vi "Constructor.vi"(6 "channel name":string, 8 "error in":errorcluster, 9 "group name":string, 10 "path":path, 11 "TDMS in":refnum<class "TDMS.lvclass">) -> (0 "error out":errorcluster, 3 "TDMS out":refnum<class "TDMS.lvclass">)   [LabVIEW 2011, in "TDMS.lvclass"]
uses:
  TDMS.lvclass
  TDMS.lvclass/TDMS.ctl
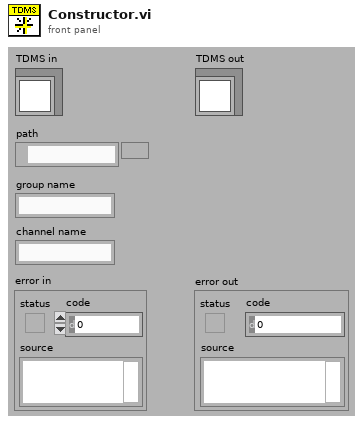
[diagram p1: front panel]
types:
  T1 = enum16{"open", "open or create", "create or replace", "create", "open (read-only)"}
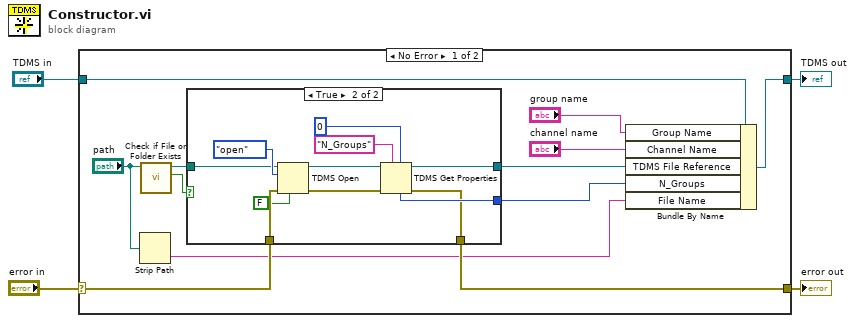
[diagram p0: block diagram]
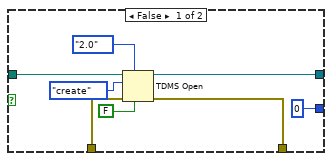
[diagram p2: hidden frame]
diagram:
  n1 = case shown="No Error" "error in" {
    selector: "error in" -> [w16 w37]
    tunnel: [w15 w37] -> w1
    tunnel: [w12 w36] -> w2
    tunnel: "TDMS in" -> [w14 w36]
    frame No Error {
      n2 = Strip Path(path="path") -> (name=w5:string)  [unwired: 1 out]
      n3 = call <vilib>:"Check if File or Folder Exists.vi"("path"="path") -> ("file or folder exists?"=w11:bool, "dup path"=w10:path)  [unwired: 8 in, 1 out]
      n4 = case shown="True" w11 {
        tunnel: w16 -> [w22 w35]
        tunnel: [w21 w26] -> w15
        tunnel: [w23 w31] -> w13
        tunnel: w10 -> [w24 w33]
        tunnel: [u16 0 w28] -> w7
        frame False {
          n5 = TDMS Open(6:FALSE ("disable buffering? (T)"), 7:enum16{"1.0", "2.0"}."2.0" ("file format version (2.0)"), 8:w22, 10:T1."create" ("operation (0:open)"), 11:w24) -> (0:w21:errorcluster, 3:w23:refnum<k34>)  [unwired: 1 in]
        }
        frame True {
          n6 = TDMS Open(6:FALSE ("disable buffering? (T)"), 8:w35, 10:T1."open" ("operation (0:open)"), 11:w33) -> (0:w27:errorcluster, 3:w32:refnum<k34>)  [unwired: 2 in]
          n7 = TDMS Get Properties(5:u16 0, 7:"N_Groups" ("property name"), 8:w27, 11:w32) -> (0:w26:errorcluster, 3:w31:refnum<k34>, 4:w28:u16)  [unwired: 2 in, 3 out]
        }
      }
      n8 = Bundle By Name(cluster=w14, "Group Name"="group name", "Channel Name"="channel name", "TDMS File Reference"=w13, "N_Groups"=w7, "File Name"=w5) -> (w12:refnum<class "TDMS.lvclass">)
    }
    frame Error {
    }
  }
  "TDMS out" <- w2
  "error out" <- w1
